vi "Oxford-IPS120-Main.vi"() -> ()   [LabVIEW 2016, in "IPS120.lvclass"]
uses:
  IPS120.lvclass
  <vilib>/JKI/JKI SMO/SMO/Typedefs/SMOState --Enum.ctl
  C:/Program Files (x86)/National Instruments/LabVIEW 2016/vi.lib/JKI/JKI SMO/SMO/SMO.lvclass
  <vilib>/JKI/JKI SMO/SMO/SMO.lvclass
panel:
  out "SMO State":T1
  out "error out":errorcluster
  in  "Stop":bool
  # "Oxford-IPS120-Main.vi"
  # "For instructions on how to use the JKI State Machine Objects, examples and video tutorials, visit:\nhttp://jki.net/state-machine-objects/\n\nJKI State Machine Objects™\nhttp://jki.net/state-machine-objects/\nCopyright (C) 2005-2015, JKI <info@jki.net>\nALL RIGHTS RESERVED"
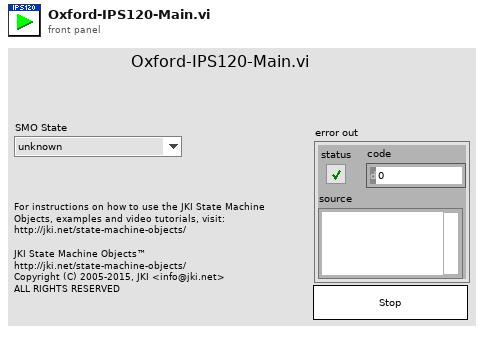
[diagram p1: front panel]
types:
  T1 = typedef "SMO.lvclass/SMOState --Enum.ctl" = enum16{"unknown", "Created", "Started", "Stopped"}
  T2 = typedef "SMO.lvclass/Public Events.ctl" = cluster{"Error":refnum<user-event>, "State":refnum<user-event>, "Reserve State":refnum<user-event>}
  T3 = cluster{"Event Registration Refnum":refnum<event-registration>}
  T4 = enum32{"Invalid", "Standard", "Closed", "Hidden", "Minimized", "Maximized"}
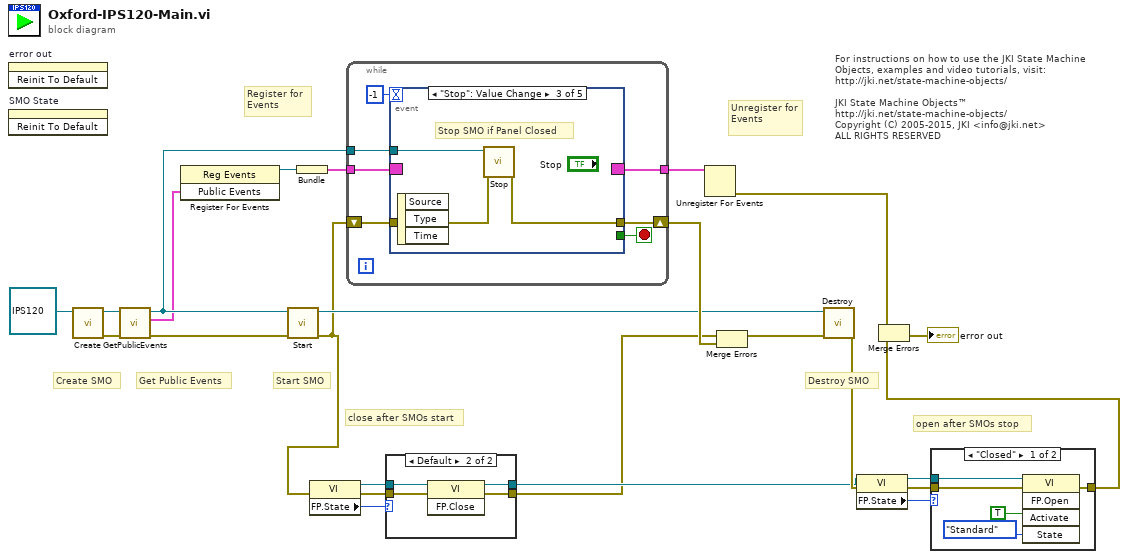
[diagram p0: block diagram]
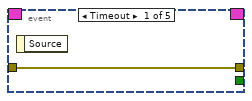
[diagram p4: hidden frame]
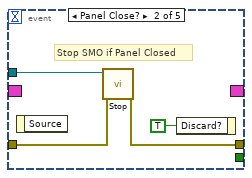
[diagram p5: hidden frame]
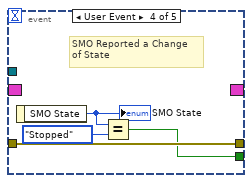
[diagram p6: hidden frame]
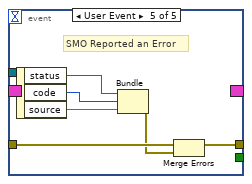
[diagram p7: hidden frame]
diagram:
  # "open after SMOs stop"
  # "close after SMOs start"
  # "For instructions on how to use the JKI State Machine Objects, examples and video tutorials, visit:\nhttp://jki.net/state-machine-objects/\n\nJKI State Machine Objects™\nhttp://jki.net/state-machine-objects/\nCopyright (C) 2005-2015, JKI <info@jki.net>\nALL RIGHTS RESERVED"
  # "Get Public Events"
  # "Start SMO"
  # "Destroy SMO"
  # "Create SMO"
  # "Unregister for Events"
  # "Register for Events"
  n1 = invoke on="error out" class="Clust (strict)" method="Reinit To Default"() -> ()  [unwired: 3 in, 3 out]
  n2 = invoke on="SMO State" class="Enum (strict)" method="Reinit To Default"() -> ()  [unwired: 3 in, 3 out]
  n3 = call <vilib>:"Create.vi"("SMO"=refnum<class "IPS120.lvclass"> refnum ("SMO.Template.lvclass")) -> ("error out"=w16:errorcluster, "SMO out"=w17:refnum<class "IPS120.lvclass">)  [unwired: 8 in, 1 out]
  n4 = call <vilib>:"GetPublicEvents.vi"("error in (no error)"=w16, "SMO"=w17) -> ("error out"=w15:errorcluster, "Public Events"=w13:T2, "SMO out"=w14:refnum<class "IPS120.lvclass">)  [unwired: 7 in]
  n5 = register-events(w13) -> (reference out=w12:refnum<event-registration>)  [unwired: 2 in, 1 out]
  n6 = call <vilib>:"Start.vi"("error in (no error)"=w15, "SMO"=w14) -> ("error out"=w3:errorcluster, "SMO out"=w18:refnum<class "IPS120.lvclass">)  [unwired: 8 in]
  n7 = Bundle("Event Registration Refnum"=w12) -> (w24:T3)  [unwired: 1 in]
  n8 = property class="VI"(error in=w3) -> (reference out=w10:refnum<vi>, error out=w9:errorcluster, "FP.State"=w11:T4)  [unwired: 1 in]
  n9 = while {
    shift-right: [w31] -> w23
    shift-left: w3 -> [w30]
    tunnel: w24 -> [w29]
    tunnel: [w28] -> w25
    tunnel: w14 -> [w27]
    stop <- w32 stop-if-true
    n10 = event shown="[2] \"Stop\": Value Change" {
      selector: w29 -> [_ _ _ _ _]
      dyn-events: [_ _ _ _ _] -> w28
      timeout: -1 -> [_ _ _ _ _]
      tunnel: [_ _ _ w41 _] -> w32
      tunnel: w27 -> [_ w37 w40 _ _]
      tunnel: [w33 w36 w39 w44 w48] -> w31
      tunnel: w30 -> [w33 w35 w38 w44 w46]
      event Timeout {
        n11 = event-data() -> ()  [unwired: 1 in, 1 out]
      }
      event Panel Close? {
        # "Stop SMO if Panel Closed"
        n12 = event-data() -> ()  [unwired: 1 in, 1 out]
        n13 = call <vilib>:"Stop.vi"("error in (no error)"=w35, "SMO"=w37) -> ("error out"=w36:errorcluster)  [unwired: 8 in, 1 out]
        n14 = event-data("Discard?"=TRUE ("OK")) -> ()  [unwired: 1 in, 1 out]
      }
      event "Stop": Value Change {
        # "Stop SMO if Panel Closed"
        n15 = event-data() -> ()  [unwired: 1 in, 3 out]
        n16 = call <vilib>:"Stop.vi"("error in (no error)"=w38, "SMO"=w40) -> ("error out"=w39:errorcluster)  [unwired: 8 in, 1 out]
      }
      event User Event {
        # "SMO Reported a Change\nof State"
        n17 = event-data() -> ("SMO State"=w43:T1)  [unwired: 1 in]
        "SMO State" <- w43
        n18 = Equal?(x=w43, y=SMOState_--Enum."Stopped") -> (x = y?=w41:bool)
      }
      event User Event {
        # "SMO Reported an Error"
        n19 = event-data() -> ("status"=w47:bool, "code"=w50:i32, "source"=w49:string)  [unwired: 1 in]
        n20 = Bundle("status"=w47, "code"=w50, "source"=w49) -> (w45:errorcluster)  [unwired: 1 in]
        n21 = Merge Errors(w46, w45) -> (w48:errorcluster)
      }
    }
  }
  n22 = case shown="Default" w11 {
    tunnel: [w52 w56] -> w2
    tunnel: w9 -> [w52 w55]
    tunnel: w10 -> [w51 w54]
    tunnel: [w51 w53] -> w4
    frame "Invalid", "Closed" {
    }
    frame Default {
      n23 = invoke class="VI" method="FP.Close"(reference=w54, error in=w55) -> (reference out=w53:refnum<vi>, error out=w56:errorcluster)  [unwired: 1 in, 1 out]
    }
  }
  n24 = Unregister For Events(event registration refnum=w25) -> (error out=w22:errorcluster)  [unwired: 1 in]
  n25 = Merge Errors(w2, w23) -> (w19:errorcluster)
  n26 = call <vilib>:"Destroy.vi"("error in (no error)"=w19, "SMO"=w18) -> ("error out"=w5:errorcluster)  [unwired: 9 in]
  n27 = property class="VI"(reference=w4, error in=w5) -> (reference out=w7:refnum<vi>, error out=w6:errorcluster, "FP.State"=w8:T4)
  n28 = case shown="\"Closed\"" w8 {
    tunnel: [w59 w62] -> w1
    tunnel: w6 -> [w58 w62]
    tunnel: w7 -> [w57 _]
    frame "Closed" {
      n29 = invoke class="VI" method="FP.Open"(reference=w57, error in=w58, "Activate"=TRUE, "State"=T4."Standard") -> (error out=w59:errorcluster)  [unwired: 1 in, 4 out]
    }
    frame Default {
    }
  }
  n30 = Merge Errors(w22, w1) -> (→"error out":errorcluster)
